vi "rszvl Configure Marker State.vi"(7 "Marker State (Off)":bool, 8 "error in (no error)":errorcluster, 9 "Marker (1)":i32=1, 10 "Channel (1)":i32=1, 11 "VISA resource name":refnum<visa-resource-name>) -> (0 "error out":errorcluster, 3 "VISA resource name out":refnum<visa-resource-name>)   [LabVIEW 2014]
doc: "This VI creates the marker numbered <Mk> and assigns it to trace no. <Ch/Tr>.\n\nAttribute(s):\nRSZVL_ATTR_NWA_MARKER_STATE\n\nRemote-control command(s):\nCALCulate<Ch/Tr>:MARKer<Mk>[:STATe] <Boolean>"
uses:
  Instance           1 36Saved   rszvl Configure Marker State .vi
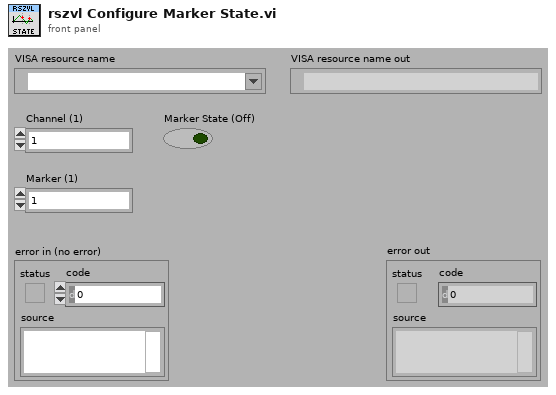
[diagram p1: front panel]
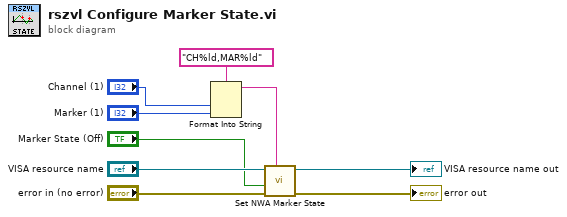
[diagram p0: block diagram]
diagram:
  n1 = Format Into String(format string="CH%ld,MAR%ld", "Channel (1)", "Marker (1)") -> (resulting string=w4:string)  [unwired: 2 in, 1 out]
  n2 = call "Set NWA Marker State"("Repeated Capabilities"=w4, "error in (no error)"="error in (no error)", "NWA Marker State (OFF)"="Marker State (Off)", "instrument handle"="VISA resource name") -> ("error out"=→"error out":errorcluster, "instrument handle out"=→"VISA resource name out":refnum<visa-resource-name>)  [unwired: 6 in]
